vi "One Hot Choice.vi"(11 "Probabilities":T1) -> (1 "hot value":dbl, 2 "hot index":u64, 3 "One hot vector":T1)   [LabVIEW 2014]
uses:
  <vilib>/Analysis/Matrix/Datatypes/RealMatrix.ctl
  <vilib>/Analysis/Matrix/NI_Matrix.lvlib
panel:
  out "max index(es)":u64[](array[numeric])
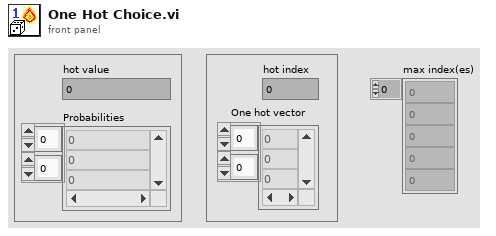
[diagram p1: front panel]
types:
  T1 = typedef "NI_Matrix.lvlib/RealMatrix.ctl" = dbl[][]
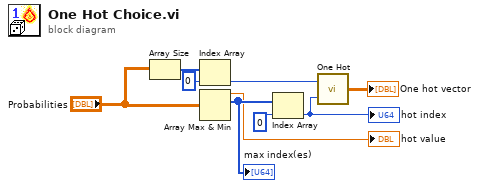
[diagram p0: block diagram]
diagram:
  n1 = Array Size(array="Probabilities") -> (size(s)=w4:i32[])
  n2 = Index Array(array=w4, index=0) -> (element=w6:i32)
  n3 = Array Max & Min(array="Probabilities") -> (max value=→"hot value":dbl, max index (indices)=w2:i32[])  [unwired: 2 out]
  "max index(es)" <- w2
  n4 = Index Array(array=w2, index=0) -> (element=w7:i32)
  "hot index" <- w7
  n5 = call "One Hot.vi"("hot index"=w7, "length"=w6) -> ("One hot vector"=→"One hot vector":T1)
